vi "Wavefroms Values from Cursors.vi"(8 "Error In":errorcluster, 9 "Waveforms In":waveform(dbl)[](array[waveform]), 11 "Waveform Graph":refnum<vi>) -> (0 "Error Out":errorcluster, 1 "Waveforms Out":waveform(dbl)[](array[waveform]), 2 "Cursor Values":dbl[][](array[numeric]))   [LabVIEW 2015]
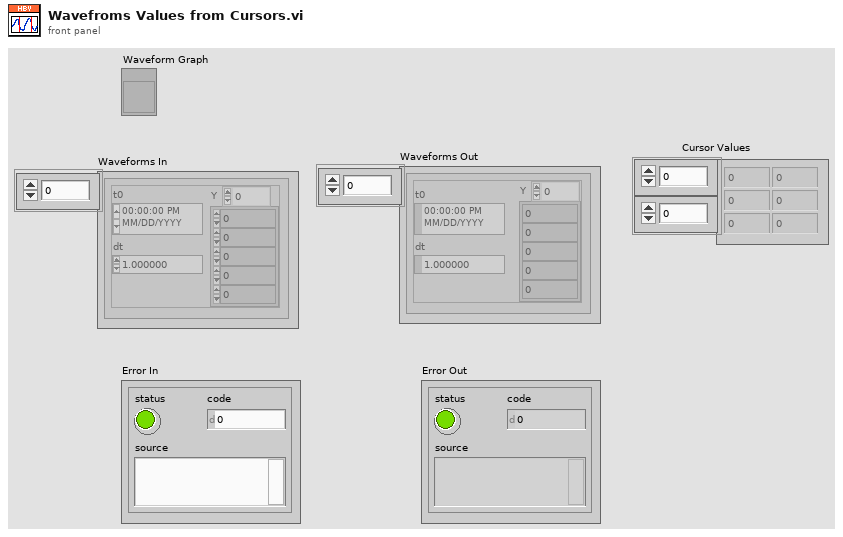
[diagram p1: front panel]
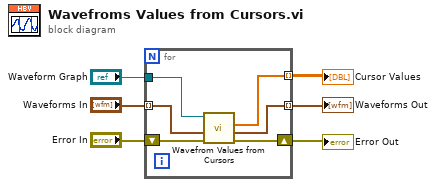
[diagram p0: block diagram]
diagram:
  n1 = for {
    shift-right: [w11] -> w4
    shift-left: "Error In" -> [w12]
    tunnel: [w10] -> w5 mode=indexing
    tunnel: "Waveforms In" -> [w9] mode=indexing
    tunnel: [w8] -> w2 mode=indexing
    tunnel: "Waveform Graph" -> [w7]
    n2 = call "Wavefrom Values from Cursors.vi"("Error In"=w12, "Waveform In"=w9, "Waveform Graph"=w7) -> ("Error Out"=w11:errorcluster, "Waveform Values"=w10:waveform(dbl), "Cursor Values"=w8:dbl[])  [unwired: 6 in]
  }
  "Error Out" <- w4
  "Cursor Values" <- w2
  "Waveforms Out" <- w5
